vi "Make VI Param(Time).vi"(1 "pTime":T1) -> (0 "Time":T2)   [LabVIEW 8.6, in "Keyence LJ-V7000.lvlib"]
uses:
  Keyence LJ-V7000.lvlib
  Public/Clusters/Time.ctl
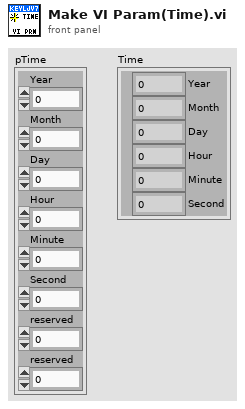
[diagram p1: front panel]
types:
  T1 = cluster{"Year":u8, "Month":u8, "Day":u8, "Hour":u8, "Minute":u8, "Second":u8, "reserved":u8, "reserved":u8}
  T2 = typedef "Keyence LJ-V7000.lvlib/Time.ctl" = cluster{"Year":u8, "Month":u8, "Day":u8, "Hour":u8, "Minute":u8, "Second":u8}
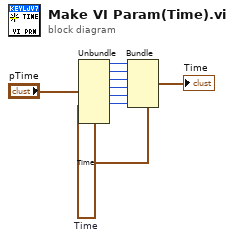
[diagram p0: block diagram]
diagram:
  w3 = T2 ?  # Time
  n1 = Unbundle("pTime") -> ("Year"=w2:u8, "Month"=w4:u8, "Day"=w5:u8, "Hour"=w6:u8, "Minute"=w7:u8, "Second"=w8:u8)  [unwired: 2 out]
  n2 = Bundle(cluster=w3, "Year"=w2, "Month"=w4, "Day"=w5, "Hour"=w6, "Minute"=w7, "Second"=w8) -> (→"Time":T2)
